vi "main.vi"() -> ()   [LabVIEW 2017, in "MediatorPatternDemo.lvclass"]
uses:
  MediatorPatternDemo.lvclass
  User Class/User.lvclass
  ConsoleOut/Print Options.ctl
panel:
  in  "User Name":u16(ring) items=["John", "Robert"]
  in  "Message":string
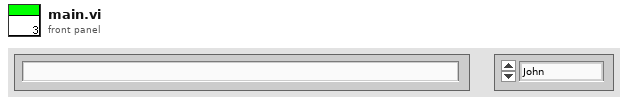
[diagram p1: front panel]
types:
  T1 = typedef "Print Options.ctl" = enum16{"Create", "Get Reference", "Print", "Print Header", "Close"}
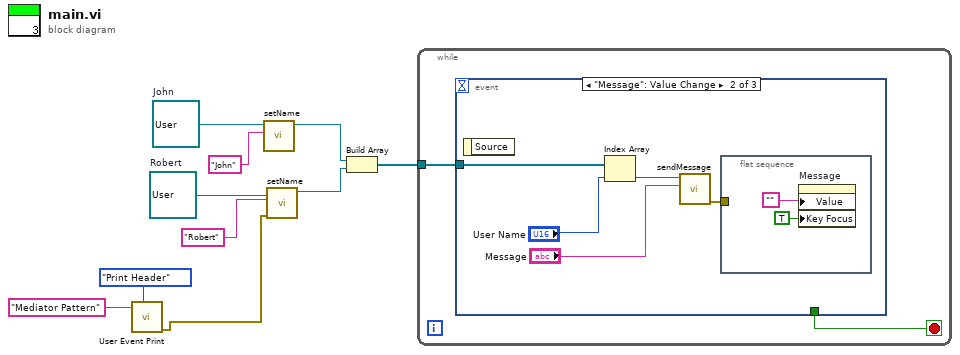
[diagram p0: block diagram]
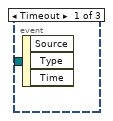
[diagram p2: hidden frame]
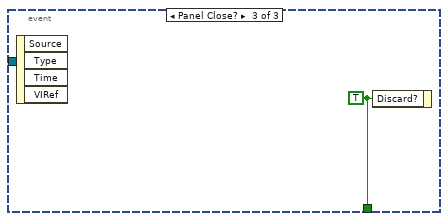
[diagram p3: hidden frame]
diagram:
  w9 = refnum<class "User.lvclass"> refnum  # Robert
  w10 = refnum<class "User.lvclass"> refnum  # John
  n1 = call "User Event Print.vi"("Options"=Print_Options."Print Header", "String to Print"="Mediator Pattern") -> ("error out"=w1:errorcluster)  [unwired: 8 in, 1 out]
  n2 = call-dynamic "setName.vi"("name"="John", "User in"=w10) -> ("User out"=w6:refnum<class "User.lvclass">)  [unwired: 8 in, 1 out]
  n3 = call-dynamic "setName.vi"("error in (no error)"=w1, "name"="Robert", "User in"=w9) -> ("User out"=w5:refnum<class "User.lvclass">)  [unwired: 7 in, 1 out]
  n4 = Build Array(w6, w5) -> (w4:refnum<class "User.lvclass">[])
  n5 = while {
    tunnel: w4 -> [w12]
    stop <- w11 stop-if-true
    n6 = event shown="[1] \"Message\": Value Change" {
      selector: _ -> [_ _ _]
      dyn-events: _ -> [_ _ _]
      timeout: _ -> [_ _ _]
      tunnel: w12 -> [_ w17 _]
      tunnel: [_ _ w20] -> w11
      event Timeout {
        n7 = event-data() -> ()  [unwired: 1 in, 3 out]
      }
      event "Message": Value Change {
        n8 = event-data() -> ()  [unwired: 1 in, 1 out]
        n9 = Index Array(array=w17, index="User Name") -> (element=w16:refnum<class "User.lvclass">)
        n10 = call-dynamic "sendMessage.vi"("Message"="Message", "User in"=w16) -> ("error out"=w14:errorcluster)  [unwired: 8 in, 1 out]
        n11 = flat-sequence {
          tunnel: w14 -> [_]
          frame #0 {
            n12 = property on="Message" class="Str"("Value"="", "Key Focus"=TRUE) -> ()  [unwired: 2 in, 2 out]
          }
        }
      }
      event Panel Close? {
        w20 = TRUE ("Discard?")
        n13 = event-data() -> ()  [unwired: 1 in, 4 out]
        n14 = event-data("Discard?"=w20) -> ()  [unwired: 1 in, 1 out]
      }
    }
  }
